vi "Initilaize Views.vi"(8 "error in (no error)":errorcluster, 11 "Example Controller in":refnum<class "Example Controller.lvclass">) -> (0 "error out":errorcluster, 3 "Example Controller out":refnum<class "Example Controller.lvclass">)   [LabVIEW 2023, in "Example MVC Actors.lvlib" / "Example Controller.lvlib" / "Example Controller.lvclass"]
uses:
  Example Controller.lvclass
  Example Controller.lvclass/Example Controller.ctl
  View/View.lvclass/View.ctl
  View/properties/Write Name.vi
  Controller/Controller.lvclass
  View/View.lvclass
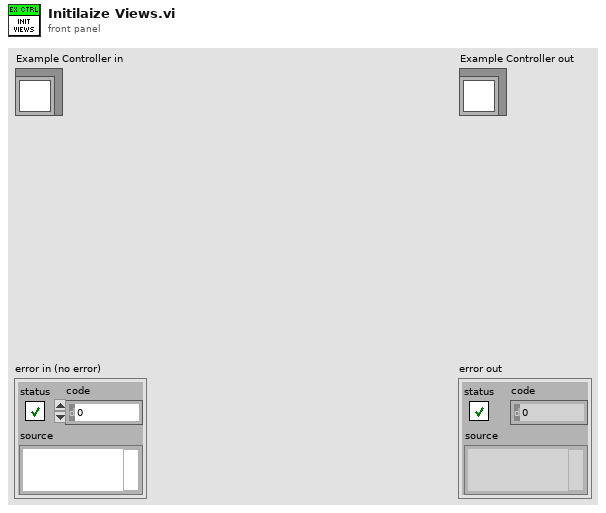
[diagram p1: front panel]
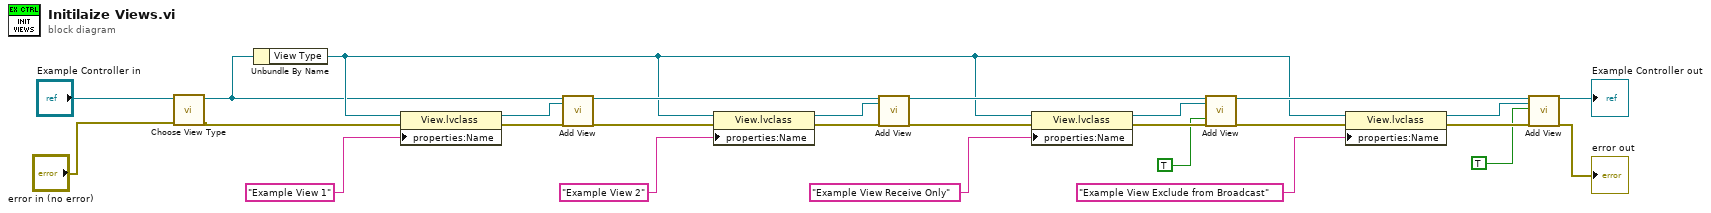
[diagram p0: block diagram]
diagram:
  n1 = call-dynamic "Choose View Type.vi"("error in (no error)"="error in (no error)", "Example Controller Actor in"="Example Controller in") -> ("error out"=w3:errorcluster, "Example Controller Actor out"=w4:refnum<class "Example Controller.lvclass">)  [unwired: 8 in]
  n2 = Unbundle By Name(w4) -> ("View Type"=w5:refnum<class "View.lvclass">)
  n3 = property class="View.lvclass"(reference=w5, error in=w3, "properties:Name"="Example View 1" ("Debug Alias")) -> (reference out=w27:refnum<class "View.lvclass">, error out=w25:errorcluster)
  n4 = call "Add View.vi"("Controller in"=w4, "View Actor"=w27, "error in (no error)"=w25) -> ("Controller out"=w24:refnum<class "Example Controller.lvclass">, "error out"=w18:errorcluster)  [unwired: 14 in, 1 out]
  n5 = property class="View.lvclass"(reference=w5, error in=w18, "properties:Name"="Example View 2" ("Debug Alias")) -> (reference out=w20:refnum<class "View.lvclass">, error out=w17:errorcluster)
  n6 = call "Add View.vi"("Controller in"=w24, "View Actor"=w20, "error in (no error)"=w17) -> ("Controller out"=w23:refnum<class "Example Controller.lvclass">, "error out"=w16:errorcluster)  [unwired: 14 in, 1 out]
  n7 = property class="View.lvclass"(reference=w5, error in=w16, "properties:Name"="Example View Receive Only" ("Debug Alias")) -> (reference out=w19:refnum<class "View.lvclass">, error out=w15:errorcluster)
  n8 = call "Add View.vi"("Controller in"=w23, "View Actor"=w19, "Receive Only (F)"=TRUE, "error in (no error)"=w15) -> ("Controller out"=w10:refnum<class "Example Controller.lvclass">, "error out"=w9:errorcluster)  [unwired: 13 in, 1 out]
  n9 = property class="View.lvclass"(reference=w5, error in=w9, "properties:Name"="Example View Exclude from Broadcast" ("Debug Alias")) -> (reference out=w12:refnum<class "View.lvclass">, error out=w11:errorcluster)
  n10 = call "Add View.vi"("Controller in"=w10, "View Actor"=w12, "Exclude From Broadcast (F)"=TRUE, "error in (no error)"=w11) -> ("Controller out"=→"Example Controller out":refnum<class "Example Controller.lvclass">, "error out"=→"error out":errorcluster)  [unwired: 13 in, 1 out]
